vi "Init.vi"(7 "Name Delimiter (.)":string=".", 8 "error in (no error)":errorcluster, 11 "INI Path":path) -> (0 "error out":errorcluster, 3 "Config-INI out":refnum<class "Config-INI.lvclass">)   [LabVIEW 2020, in "CDM-Config.lvlib" / "Config-INI.lvclass"]
uses:
  Config-INI.lvclass
  Config-INI.lvclass/Config-INI.ctl
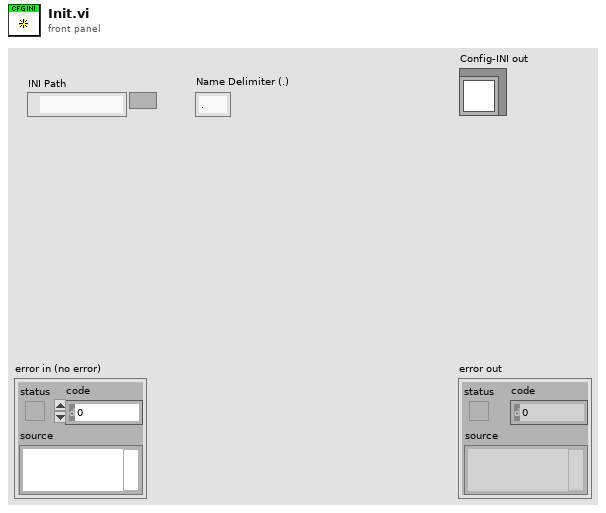
[diagram p1: front panel]
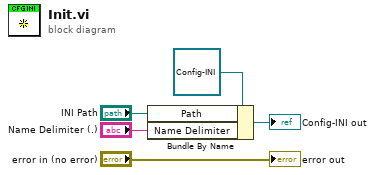
[diagram p0: block diagram]
diagram:
  n1 = Bundle By Name(cluster=refnum<class "Config-INI.lvclass"> refnum ("Config-INI in"), "Path"="INI Path", "Name Delimiter"="Name Delimiter (.)") -> (→"Config-INI out":refnum<class "Config-INI.lvclass">)
  "error out" <- "error in (no error)"
